vi "Generic command handler.vi"(8 "error in (no error)":errorcluster, 10 "Message in":refnum<class "GenericMessage.lvclass">, 11 "focus in":refnum<class "focus.lvclass">) -> (0 "error out":errorcluster, 2 "value":string, 3 "focus out":refnum<class "focus.lvclass">)   [LabVIEW 2012, in "focus.lvclass"]
doc: "The generic_command_handler processes the command 'generic'. Commands which are not part of the predefined list of commands fall under the 'generic' command for special activity."
uses:
  focus.lvclass
  <vilib>/Distrio/Murmex/GenericMessage/GenericMessage.lvclass
  <vilib>/Distrio/Murmex/Murmex/Murmex.lvclass
  focus.lvclass/focus.ctl
  <vilib>/Distrio/Murmex/ProceedMessage/ProceedMessage.lvclass
  <vilib>/Distrio/Murmex/Message/Message.lvclass
panel:
  # "This method is called when the GENERIC\ntrigger is sent. \n\nOverride this method when your component needs to\nrespond to this trigger. \n\nCall parent for proper implementation"
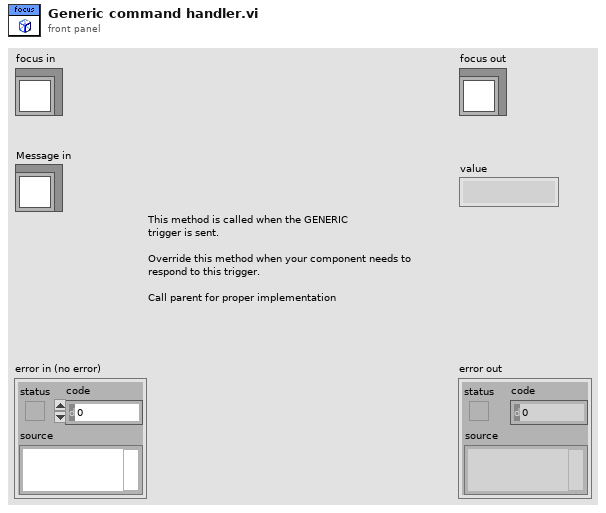
[diagram p1: front panel]
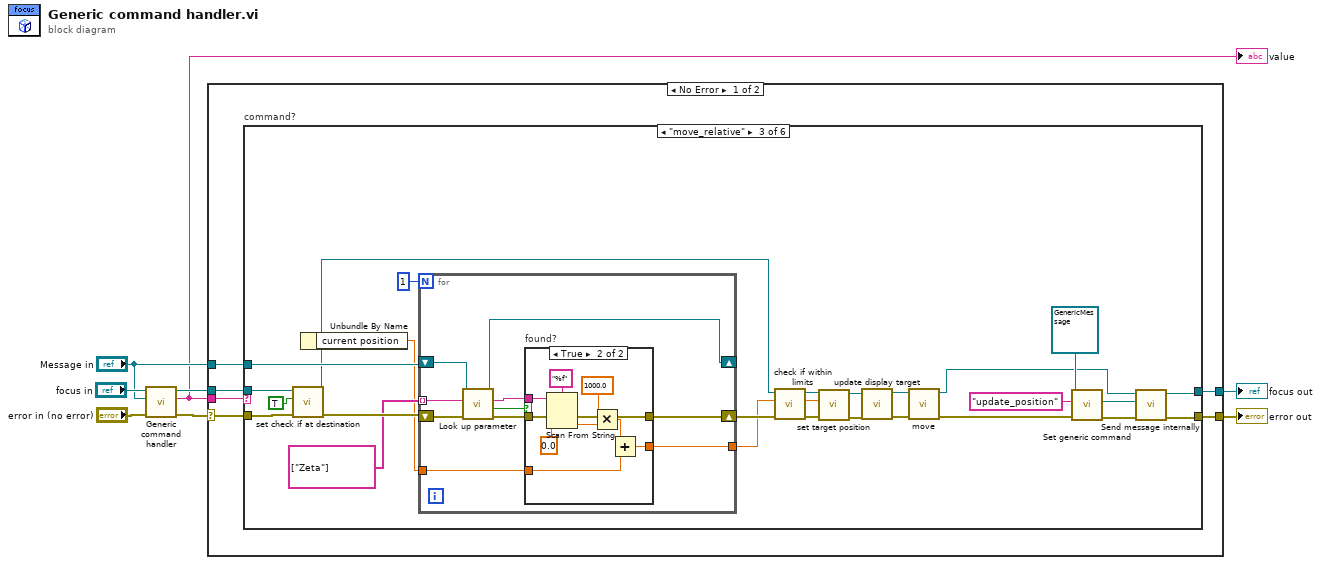
[diagram p0: block diagram]
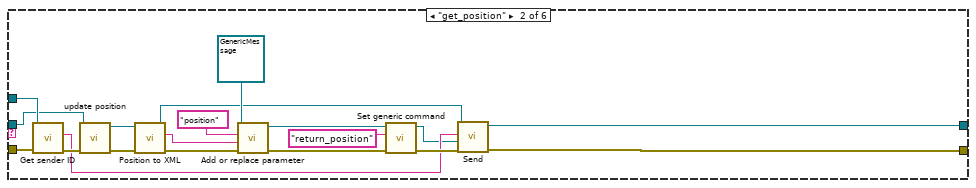
[diagram p3: hidden frame]
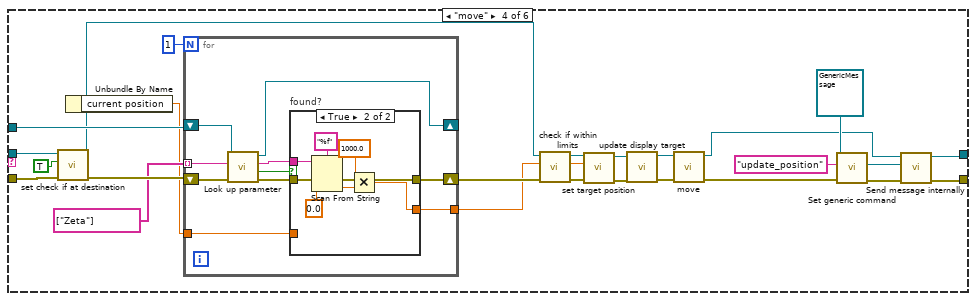
[diagram p5: hidden frame]
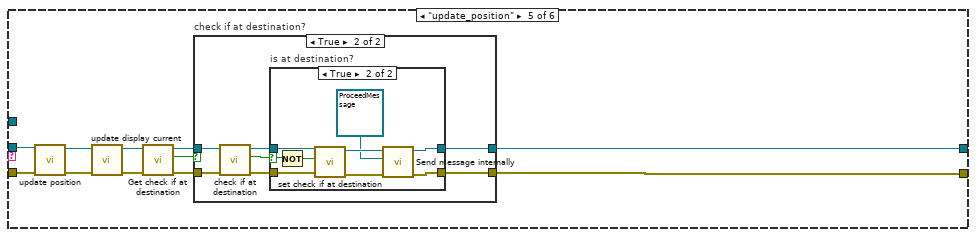
[diagram p7: hidden frame]
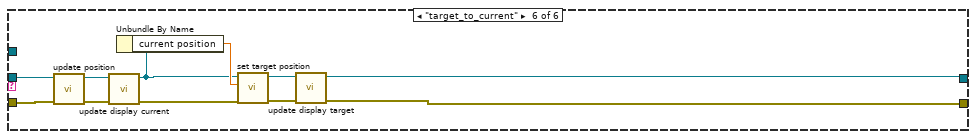
[diagram p10: hidden frame]
diagram:
  n1 = call-parent "Generic command handler.vi"("error in (no error)"="error in (no error)", "Message in"="Message in", "Murmex in"="focus in") -> ("error out"=w6:errorcluster, "value"=w1:string, "Murmex out"=w5:refnum<class "focus.lvclass">)  [unwired: 6 in]
  "value" <- w1
  n2 = case shown="No Error" w6 {
    selector: w6 -> [w14 w172]
    tunnel: w1 -> [w13 _]
    tunnel: w5 -> [w12 w173]
    tunnel: "Message in" -> [w11 _]
    tunnel: [w10 w172] -> w3
    tunnel: [w9 w173] -> w2
    frame No Error {
      n3 = case "command?" shown="\"move_relative\"" w13 {
        tunnel: w14 -> [w15 w35 w61 w109 w140 w171]
        tunnel: w12 -> [w16 w30 w59 w107 w132 w163]
        tunnel: w11 -> [_ w31 w56 w104 _ _]
        tunnel: [w15 w22 w39 w87 w133 w164] -> w10
        tunnel: [w16 w20 w36 w84 w130 w161] -> w9
        frame Default {
        }
        frame "get_position" {
          n4 = call <vilib>:"Get sender ID.vi"("error in (no error)"=w35, "Message in"=w31) -> ("error out"=w32:errorcluster, "sender"=w19:string)  [unwired: 7 in, 1 out]
          n5 = call-dynamic "update position.vi"("error in (no error)"=w32, "focus in"=w30) -> ("error out"=w34:errorcluster, "focus out"=w33:refnum<class "focus.lvclass">)  [unwired: 8 in]
          n6 = call-dynamic "Position to XML.vi"("error in (no error)"=w34, "focus in"=w33) -> ("error out"=w27:errorcluster, "XML string"=w17:string, "focus out"=w21:refnum<class "focus.lvclass">)  [unwired: 7 in]
          n7 = call <vilib>:"Add or replace parameter.vi"("error in (no error)"=w27, "value"=w17, "name"="position", "Message in"=refnum<class "GenericMessage.lvclass"> refnum ("Distrio Murmex 1.1:GenericMessage")) -> ("error out"=w25:errorcluster, "Message out"=w24:refnum<class "GenericMessage.lvclass">)  [unwired: 6 in]
          n8 = call <vilib>:"Set generic command.vi"("error in (no error)"=w25, "generic command"="return_position", "GenericMessage in"=w24) -> ("error out"=w23:errorcluster, "GenericMessage out"=w18:refnum<class "GenericMessage.lvclass">)  [unwired: 7 in]
          n9 = call <vilib>:"Send.vi"("error in (no error)"=w23, "Message"=w18, "recipient"=w19, "Murmex in"=w21) -> ("error out"=w22:errorcluster, "Murmex out"=w20:refnum<class "focus.lvclass">)  [unwired: 6 in]
        }
        frame "move_relative" {
          n10 = call-dynamic "set check if at destination.vi"("error in (no error)"=w61, "check if at destination"=TRUE, "focus in"=w59) -> ("error out"=w58:errorcluster, "focus out"=w45:refnum<class "focus.lvclass">)  [unwired: 7 in]
          n11 = Unbundle By Name(w45) -> ("current position"=w54:dbl)
          n12 = for {
            N: 1 -> [_]
            shift-right: [w68] -> w53
            shift-left: w58 -> [w71]
            tunnel: string[] ["Zeta"] -> [w62] mode=indexing
            shift-right: [w65] -> _
            shift-left: w56 -> [w66]
            tunnel: w54 -> [w64]
            tunnel: [w63] -> w44
            n13 = call <vilib>:"Look up parameter.vi"("error in (no error)"=w71, "name"=w62, "Message in"=w66) -> ("error out"=w70:errorcluster, "found?"=w69:bool, "key"=w67:string, "Message out"=w65:refnum<class "GenericMessage.lvclass">)  [unwired: 5 in]
            n14 = case "found?" shown="True" w69 {
              tunnel: w70 -> [w73 w83]
              tunnel: [w73 w77] -> w68
              tunnel: w67 -> [_ w81]
              tunnel: [w72 w79] -> w63
              tunnel: w64 -> [w72 w78]
              frame False {
              }
              frame True {
                n15 = Scan From String(format string="%f", input string=w81, error in=w83, default 1=0.0 ("default value 1")) -> (error out=w77:errorcluster, output 1=w75:dbl)  [unwired: 1 in, 2 out]
                n16 = Multiply(x=1000.0, y=w75) -> (x*y=w76:dbl)
                n17 = Add(x=w76, y=w78) -> (x+y=w79:dbl)
              }
            }
          }
          n18 = call-dynamic "check if within limits.vi"("error in (no error)"=w53, "Numeric"=w44, "focus in"=w45) -> ("error out"=w52:errorcluster, "approved position"=w51:dbl, "focus out"=w50:refnum<class "focus.lvclass">)  [unwired: 5 in, 1 out]
          n19 = call-dynamic "set target position.vi"("error in (no error)"=w52, "target position"=w51, "focus in"=w50) -> ("error out"=w49:errorcluster, "focus out"=w48:refnum<class "focus.lvclass">)  [unwired: 7 in]
          n20 = call-dynamic "update display target.vi"("error in (no error)"=w49, "focus in"=w48) -> ("error out"=w47:errorcluster, "focus out"=w46:refnum<class "focus.lvclass">)  [unwired: 8 in]
          n21 = call-dynamic "move.vi"("error in (no error)"=w47, "focus in"=w46) -> ("error out"=w38:errorcluster, "focus out"=w37:refnum<class "focus.lvclass">)  [unwired: 8 in]
          n22 = call <vilib>:"Set generic command.vi"("error in (no error)"=w38, "generic command"="update_position", "GenericMessage in"=refnum<class "GenericMessage.lvclass"> refnum ("Distrio Murmex 1.1:GenericMessage")) -> ("error out"=w40:errorcluster, "GenericMessage out"=w43:refnum<class "GenericMessage.lvclass">)  [unwired: 7 in]
          n23 = call <vilib>:"Send message internally.vi"("error in (no error)"=w40, "Message"=w43, "Murmex in"=w37) -> ("error out"=w39:errorcluster, "Murmex out"=w36:refnum<class "focus.lvclass">)  [unwired: 7 in]
        }
        frame "move" {
          n24 = call-dynamic "set check if at destination.vi"("error in (no error)"=w109, "check if at destination"=TRUE, "focus in"=w107) -> ("error out"=w106:errorcluster, "focus out"=w93:refnum<class "focus.lvclass">)  [unwired: 7 in]
          n25 = Unbundle By Name(w93) -> ("current position"=w102:dbl)
          n26 = for {
            N: 1 -> [_]
            shift-right: [w116] -> w101
            shift-left: w106 -> [w119]
            tunnel: string[] ["Zeta"] -> [w110] mode=indexing
            shift-right: [w113] -> _
            shift-left: w104 -> [w114]
            tunnel: w102 -> [w112]
            tunnel: [w111] -> w92
            n27 = call <vilib>:"Look up parameter.vi"("error in (no error)"=w119, "name"=w110, "Message in"=w114) -> ("error out"=w118:errorcluster, "found?"=w117:bool, "key"=w115:string, "Message out"=w113:refnum<class "GenericMessage.lvclass">)  [unwired: 5 in]
            n28 = case "found?" shown="True" w117 {
              tunnel: w118 -> [w121 w129]
              tunnel: [w121 w125] -> w116
              tunnel: w115 -> [_ w127]
              tunnel: [w120 w122] -> w111
              tunnel: w112 -> [w120 _]
              frame False {
              }
              frame True {
                n29 = Scan From String(format string="%f", input string=w127, error in=w129, default 1=0.0 ("default value 1")) -> (error out=w125:errorcluster, output 1=w124:dbl)  [unwired: 1 in, 2 out]
                n30 = Multiply(x=1000.0, y=w124) -> (x*y=w122:dbl)
              }
            }
          }
          n31 = call-dynamic "check if within limits.vi"("error in (no error)"=w101, "Numeric"=w92, "focus in"=w93) -> ("error out"=w100:errorcluster, "approved position"=w99:dbl, "focus out"=w98:refnum<class "focus.lvclass">)  [unwired: 5 in, 1 out]
          n32 = call-dynamic "set target position.vi"("error in (no error)"=w100, "target position"=w99, "focus in"=w98) -> ("error out"=w97:errorcluster, "focus out"=w96:refnum<class "focus.lvclass">)  [unwired: 7 in]
          n33 = call-dynamic "update display target.vi"("error in (no error)"=w97, "focus in"=w96) -> ("error out"=w95:errorcluster, "focus out"=w94:refnum<class "focus.lvclass">)  [unwired: 8 in]
          n34 = call-dynamic "move.vi"("error in (no error)"=w95, "focus in"=w94) -> ("error out"=w86:errorcluster, "focus out"=w85:refnum<class "focus.lvclass">)  [unwired: 8 in]
          n35 = call <vilib>:"Set generic command.vi"("error in (no error)"=w86, "generic command"="update_position", "GenericMessage in"=refnum<class "GenericMessage.lvclass"> refnum ("Distrio Murmex 1.1:GenericMessage")) -> ("error out"=w88:errorcluster, "GenericMessage out"=w91:refnum<class "GenericMessage.lvclass">)  [unwired: 7 in]
          n36 = call <vilib>:"Send message internally.vi"("error in (no error)"=w88, "Message"=w91, "Murmex in"=w85) -> ("error out"=w87:errorcluster, "Murmex out"=w84:refnum<class "focus.lvclass">)  [unwired: 7 in]
        }
        frame "update_position" {
          n37 = call-dynamic "update position.vi"("error in (no error)"=w140, "focus in"=w132) -> ("error out"=w139:errorcluster, "focus out"=w138:refnum<class "focus.lvclass">)  [unwired: 8 in]
          n38 = call-dynamic "update display current.vi"("error in (no error)"=w139, "focus in"=w138) -> ("error out"=w137:errorcluster, "focus out"=w136:refnum<class "focus.lvclass">)  [unwired: 8 in]
          n39 = call-dynamic "Get check if at destination.vi"("error in (no error)"=w137, "focus in"=w136) -> ("error out"=w134:errorcluster, "check if at destination"=w135:bool, "focus out"=w131:refnum<class "focus.lvclass">)  [unwired: 7 in]
          n40 = case "check if at destination?" shown="True" w135 {
            tunnel: w134 -> [w141 w149]
            tunnel: [w141 w146] -> w133
            tunnel: w131 -> [w142 w145]
            tunnel: [w142 w143] -> w130
            frame False {
            }
            frame True {
              n41 = call-dynamic "check if at destination.vi"("error in (no error)"=w149, "focus in"=w145) -> ("error out"=w147:errorcluster, "at destination?"=w148:bool, "focus out"=w144:refnum<class "focus.lvclass">)  [unwired: 7 in]
              n42 = case "is at destination?" shown="True" w148 {
                selector: w148 -> [_ w160]
                tunnel: w147 -> [w150 w158]
                tunnel: [w150 w156] -> w146
                tunnel: w144 -> [w151 w155]
                tunnel: [w151 w152] -> w143
                frame False {
                }
                frame True {
                  n43 = Not(x=w160) -> (.not. x?=w159:bool)
                  n44 = call-dynamic "set check if at destination.vi"("error in (no error)"=w158, "check if at destination"=w159, "focus in"=w155) -> ("error out"=w157:errorcluster, "focus out"=w154:refnum<class "focus.lvclass">)  [unwired: 7 in]
                  n45 = call <vilib>:"Send message internally.vi"("error in (no error)"=w157, "Message"=refnum<class "ProceedMessage.lvclass"> refnum ("Distrio Murmex 1.1:ProceedMessage"), "Murmex in"=w154) -> ("error out"=w156:errorcluster, "Murmex out"=w152:refnum<class "focus.lvclass">)  [unwired: 7 in]
                }
              }
            }
          }
        }
        frame "target_to_current" {
          n46 = call-dynamic "update position.vi"("error in (no error)"=w171, "focus in"=w163) -> ("error out"=w170:errorcluster, "focus out"=w169:refnum<class "focus.lvclass">)  [unwired: 8 in]
          n47 = call-dynamic "update display current.vi"("error in (no error)"=w170, "focus in"=w169) -> ("error out"=w167:errorcluster, "focus out"=w162:refnum<class "focus.lvclass">)  [unwired: 8 in]
          n48 = Unbundle By Name(w162) -> ("current position"=w168:dbl)
          n49 = call-dynamic "set target position.vi"("error in (no error)"=w167, "target position"=w168, "focus in"=w162) -> ("error out"=w166:errorcluster, "focus out"=w165:refnum<class "focus.lvclass">)  [unwired: 7 in]
          n50 = call-dynamic "update display target.vi"("error in (no error)"=w166, "focus in"=w165) -> ("error out"=w164:errorcluster, "focus out"=w161:refnum<class "focus.lvclass">)  [unwired: 8 in]
        }
      }
    }
    frame Error {
    }
  }
  "error out" <- w3
  "focus out" <- w2
